vi "day 20 task 1 array.vi"() -> ()   [LabVIEW 2019]
panel:
  out "result":i32
  out "sequence of moves":i32[][](array[numeric])
  out "final positions":i32[](array[numeric])
  # "Initial arrangement:\n1, 2, -3, 3, -2, 0, 4\n\n\n\n\n1 moves between 2 and -3:\n2, 1, -3, 3, -2, 0, 4\n\n\n\n\n2 moves between -3 and 3:\n1, -3, 2, 3, -2, 0, 4\n\n\n-3 moves between -2 and 0:\n1, 2, 3, -2, -3, 0, 4\n\n\n\n\n3 moves between 0 and 4:\n1, 2, -2, -3, 0, 3, 4\n\n\n\n-2 moves between 4 and 1:\n1, 2, -3, 0, 3, 4, -2\n\n\n\n\n0 does not move:\n1, 2, -3, 0, 3, 4, -2\n\n\n\n4 moves between -3 and 0:\n1, 2, -3, 4, 0, 3, -2"
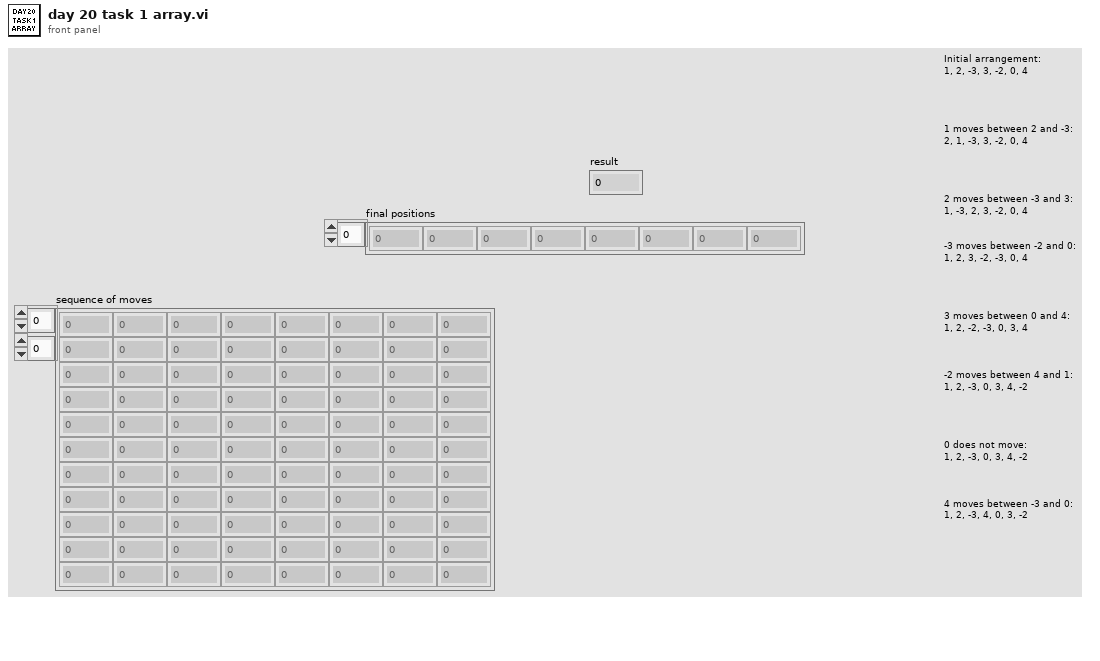
[diagram p1: front panel]
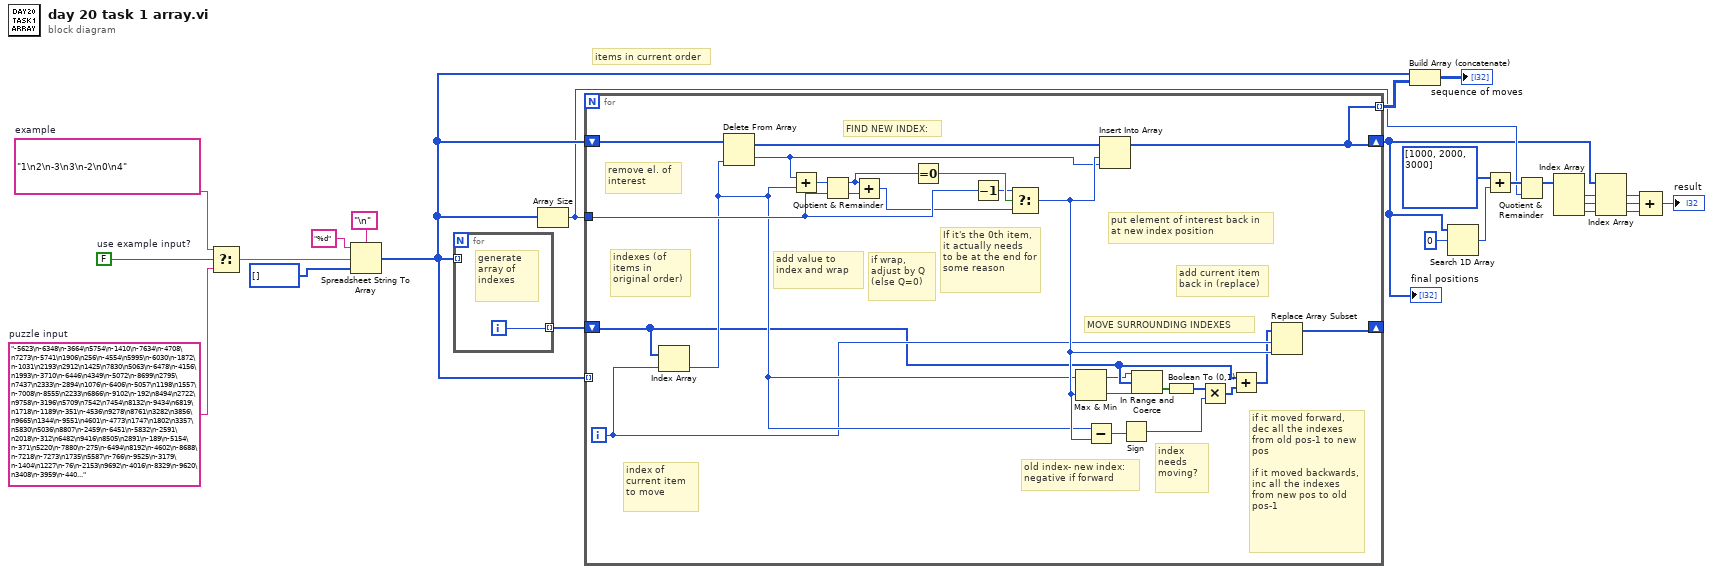
[diagram p0: block diagram]
diagram:
  w20 = FALSE  # use example input?
  w21 = "-5623\n-6348\n-3664\n5754\n-1410\n-7634\n-4708\n7273\n-5741\n1906\n256\n-4554\n5995\n-6030\n-1872\n-1031\n2193\n2912\n1425\n7830\n5063\n-6478\n-4156\n1993\n-3710\n-6446\n4349\n-5072\n-8699\n2795\n7437\n2333\n-2894\n1076\n-6406\n-5057\n1198\n1557\n-7008\n-8555\n2233\n6866\n-9102\n-192\n8494\n2722\n9758\n-3196\n5709\n7542\n7454\n8132\n-9434\n6819\n1718\n-1189\n-351\n-4536\n9278\n8761\n3282\n3856\n9665\n1344\n-9551\n4601\n-4773\n1747\n1802\n3357\n5830\n5036\n8807\n-2459\n-6451\n-5832\n-2591\n2018\n-312\n6482\n9416\n8505\n2891\n-189\n-5154\n-371\n5220\n-7880\n-275\n-6494\n8192\n-4602\n-8688\n-7218\n-7273\n1735\n5587\n-766\n-9525\n-3179\n-1404\n1227\n-76\n-2153\n9692\n-4016\n-8329\n-9620\n3408\n-3959\n-440..."  # puzzle input
  w22 = "1\n2\n-3\n3\n-2\n0\n4"  # example
  # "items in current order"
  n1 = Select(t=w22, s=w20, f=w21) -> (s? t:f=w19:string)
  n2 = Spreadsheet String To Array(delimiter (Tab)="\n", format string="%d", spreadsheet string=w19, array type (2D Dbl)=i32[] []) -> (array=w17:i32[])
  n3 = for {
    tunnel: w17 -> [_] mode=indexing
    tunnel: [w26] -> w18 mode=indexing
    i -> [w26]
    # "generate array of indexes"
  }
  n4 = Array Size(array=w17) -> (size(s)=w10:i32)
  n5 = for {
    tunnel: w17 -> [_] mode=indexing
    shift-right: [w48] -> _
    shift-left: w18 -> [w40]
    shift-right: [w49] -> w5
    shift-left: w17 -> [w43]
    tunnel: w10 -> [w47]
    tunnel: [w49] -> w16 mode=indexing
    i -> [w41]
    # "if it moved forward, dec all the indexes from old pos-1 to new pos\n\nif it moved backwards, inc all the indexes from new pos to old pos-1"
    # "index needs moving?"
    # "MOVE SURROUNDING INDEXES"
    # "add current item\nback in (replace)"
    # "put element of interest back in\nat new index position"
    # "FIND NEW INDEX:"
    # "If it's the 0th item, it actually needs\nto be at the end for some reason"
    # "if wrap, adjust by Q\n(else Q=0)"
    # "add value to index and wrap"
    # "old index- new index:\nnegative if forward"
    # "index of current item to move"
    # "remove el. of \ninterest"
    # "indexes (of items in original order)"
    n6 = Index Array(array=w40, index=w41) -> (element=w42:i32)
    n7 = Delete From Array(array=w43, index=w42) -> (deleted portion=w44:i32, array with subset deleted=w50:i32[])  [unwired: 1 in]
    n8 = Add(x=w44, y=w42) -> (x+y=w39:i32)
    n9 = Quotient & Remainder(x=w39, y=w47) -> (x-y*floor(x/y)=w30:i32, floor(x/y)=w27:i32)
    n10 = Add(x=w30, y=w27) -> (x+y=w28:i32)
    n11 = Equal To 0?(x=w30) -> (x = 0?=w45:bool)
    n12 = Decrement(x=w47) -> (x-1=w29:i32)
    n13 = Select(t=w29, s=w45, f=w28) -> (s? t:f=w46:i32)
    n14 = Max & Min(x=w42, y=w46) -> (max(x,y)=w38:i32, min(x,y)=w37:i32)
    n15 = Subtract(x=w42, y=w46) -> (x-y=w36:i32)
    n16 = Insert Into Array(array=w50, index=w46, new element=w44) -> (w49:i32[])
    n17 = Sign(1:w36) -> (0:w33:i32)
    n18 = In Range and Coerce(upper limit=w38, x=w40, lower limit=w37) -> (In Range?=w35:bool[])  [unwired: 1 out]
    n19 = Boolean To (0,1)(Boolean=w35) -> (0, 1=w34:i16[])
    n20 = Multiply(x=w34, y=w33) -> (x*y=w32:i32[])
    n21 = Add(x=w40, y=w32) -> (x+y=w31:i32[])
    n22 = Replace Array Subset(array=w31, new element=w46, index=w41) -> (w48:i32[])
  }
  "final positions" <- w5
  n23 = Build Array (concatenate)(w17, w16) -> (→"sequence of moves":i32[][])
  n24 = Search 1D Array(1D array=w5, element=0) -> (index of element=w13:i32)  [unwired: 1 in]
  n25 = Add(x=i32[] [1000, 2000, 3000], y=w13) -> (x+y=w11:i32[])
  n26 = Quotient & Remainder(x=w11, y=w10) -> (x-y*floor(x/y)=w9:i32[])  [unwired: 1 out]
  n27 = Index Array(array=w9) -> (element #1=w8:i32, element #2=w7:i32, element #3=w6:i32)  [unwired: 3 in]
  n28 = Index Array(array=w5, index #1=w8, index #2=w7, index #3=w6) -> (element #1=w4:i32, element #2=w3:i32, element #3=w2:i32)
  n29 = Compound Arithmetic op=ADD(w4, w3, w2) -> (→"result":i32)
